vi "Generate Broadcast Message.vi"(8 "error in (no error)":errorcluster, 9 "Message Data":variant, 10 "Message":string, 11 "Mock Process In":refnum<class "Mock Process.lvclass">) -> (0 "error out":errorcluster, 3 "Mock Process Out":refnum<class "Mock Process.lvclass">)   [LabVIEW 2020, in "Mock Process.lvclass"]
uses:
  Mock Process.lvclass
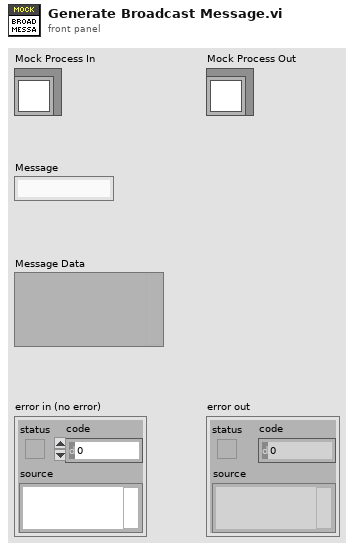
[diagram p1: front panel]
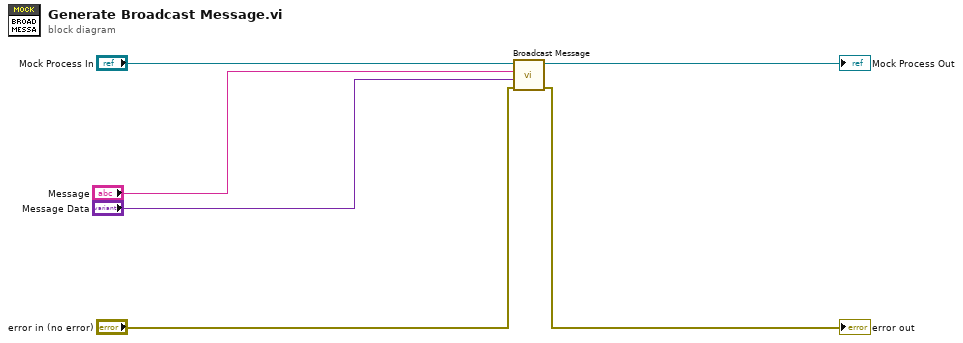
[diagram p0: block diagram]
diagram:
  n1 = call-dynamic "Broadcast Message.vi"("error in (no error)"="error in (no error)", "Message Data"="Message Data", "Message"="Message", "Rig Process In"="Mock Process In") -> ("error out"=→"error out":errorcluster, "Rig Process Out"=→"Mock Process Out":refnum<class "Mock Process.lvclass">)  [unwired: 6 in]
